vi "dbc-destructor.vi"(8 "error in (no error)":errorcluster, 11 "dbc in":refnum<class "dbc.lvclass">) -> (0 "error out":errorcluster)   [LabVIEW 2015, in "dbc.lvclass"]
uses:
  dbc.lvclass
  dbc.lvclass/dbc.ctl
  class.bFrameIO/bFrameIO.lvclass
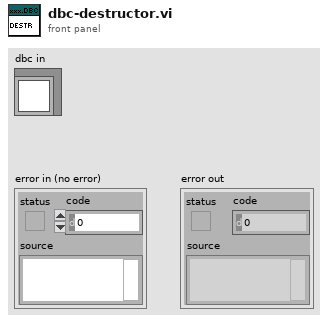
[diagram p1: front panel]
types:
  T1 = typedef "dbc-file-data.ctl" = cluster{"dbc.ref":refnum<k21>, "dbc.file":path, "alias":string}
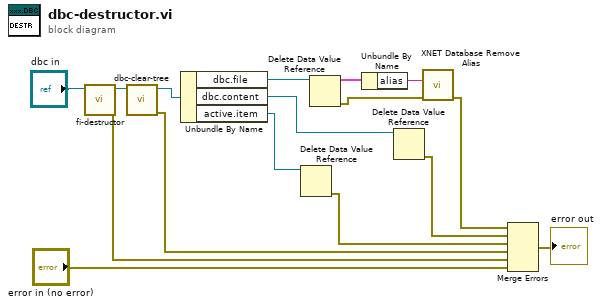
[diagram p0: block diagram]
diagram:
  n1 = call "fi-destructor.vi"("frameInput in"="dbc in") -> ("error out"=w5:errorcluster, "frameInput out"=w6:refnum<class "dbc.lvclass">)  [unwired: 9 in]
  n2 = call "dbc-clear-tree.vi"("dbc in"=w6) -> ("error out"=w3:errorcluster, "dbc out"=w4:refnum<class "dbc.lvclass">)  [unwired: 9 in]
  n3 = Unbundle By Name(w4) -> ("dbc.file"=w11:refnum<data-value>, "dbc.content"=w8:refnum<data-value>, "active.item"=w2:refnum<data-value>)
  n4 = Delete Data Value Reference(data value reference=w2) -> (error out=w1:errorcluster)  [unwired: 1 in, 1 out]
  n5 = Delete Data Value Reference(data value reference=w11) -> (data value=w10:T1, error out=w13:errorcluster)  [unwired: 1 in]
  n6 = Unbundle By Name(w10) -> ("alias"=w9:string)
  n7 = Delete Data Value Reference(data value reference=w8) -> (error out=w7:errorcluster)  [unwired: 1 in, 1 out]
  n8 = call <vilib>:"XNET Database Remove Alias.vi"("alias"=w9, "error in (no error)"=w13) -> ("error out"=w14:errorcluster)  [unwired: 13 in]
  n9 = Merge Errors(w14, w7, w1, w3, w5, "error in (no error)") -> (→"error out":errorcluster)
